vi "Intan_ADC_Calibrate.vi"(3 "error in":errorcluster, 5 "VISA resource name":refnum<visa-resource-name>="COM1") -> (0 "error out":errorcluster, 1 "Text response":string, 2 "VISA resource name out":refnum<visa-resource-name>)   [LabVIEW 2017]
doc: "Use this VI to perform ADC self-calibration. This should be called AFTER configuring filters (and other registers)."
panel:
  in  "Teensy event char":string="a"
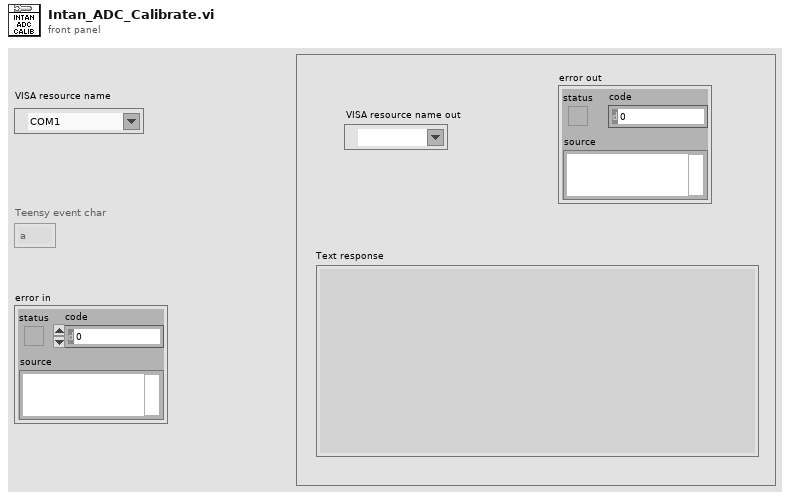
[diagram p1: front panel]
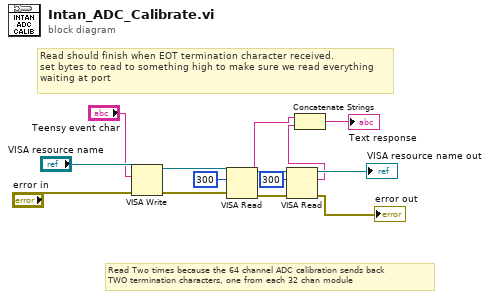
[diagram p0: block diagram]
diagram:
  # "Read Two times because the 64 channel ADC calibration sends back\nTWO termination characters, one from each 32 chan module"
  # "Read should finish when EOT termination character received. \nset bytes to read to something high to make sure we read everything waiting at port"
  n1 = VISA Write(VISA resource name="VISA resource name", write buffer="Teensy event char", error in (no error)="error in") -> (VISA resource name out=w11:refnum<visa-resource-name>, error out=w10:errorcluster)  [unwired: 1 out]
  n2 = VISA Read(VISA resource name=w11, byte count=u32 300, error in (no error)=w10) -> (VISA resource name out=w8:refnum<visa-resource-name>, read buffer=w4:string, error out=w6:errorcluster)  [unwired: 1 out]
  n3 = VISA Read(VISA resource name=w8, byte count=u32 300, error in (no error)=w6) -> (VISA resource name out=→"VISA resource name out":refnum<visa-resource-name>, read buffer=w3:string, error out=→"error out":errorcluster)  [unwired: 1 out]
  n4 = Concatenate Strings(w4, w3) -> (→"Text response":string)
